vi "TidyOverlappingWires.vi"(8 "Error In":errorcluster, 10 "New case structure ref":refnum<vi>, 11 "VI ref in":refnum<vi>) -> (0 "Error Out":errorcluster)   [LabVIEW 2017, in "ErrorStructureDrawer.lvlib"]
doc: "Clean wires that are at risk of overlapping others as a result of the actions of the plugin.\n\nNote that this acts on wires that this VI thinks are \"at risk\" of overlap as there is no obvious method to directly check if wires overlap."
uses:
  ErrorStructureDrawer.lvlib
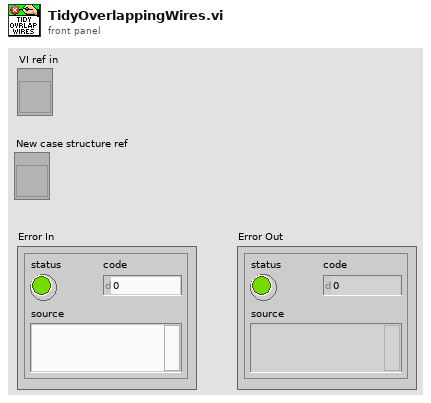
[diagram p1: front panel]
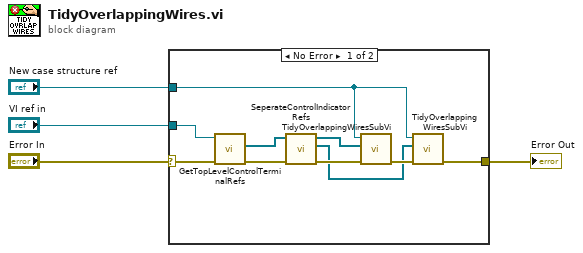
[diagram p0: block diagram]
diagram:
  n1 = case shown="No Error" "Error In" {
    selector: "Error In" -> [w6 w15]
    tunnel: "VI ref in" -> [w11 _]
    tunnel: "New case structure ref" -> [w9 _]
    tunnel: [w5 w15] -> w1
    frame No Error {
      n2 = call "GetTopLevelControlTerminalRefs.vi"("error in (no error)"=w6, "VI ref in"=w11) -> ("error out"=w13:errorcluster, "Control terminals on top-level"=w14:refnum<vi>[])  [unwired: 7 in, 1 out]
      n3 = call "SeperateControlIndicatorRefs.vi"("error in (no error)"=w13, "Terminal references"=w14) -> ("error out"=w12:errorcluster, "Indicator references"=w7:refnum<vi>[], "Control references"=w10:refnum<vi>[])  [unwired: 7 in]
      n4 = call "TidyOverlappingWiresSubVi.vi"("Error In"=w12, "Control references"=w10, "New case structure ref"=w9) -> ("Error Out"=w8:errorcluster)  [unwired: 8 in]
      n5 = call "TidyOverlappingWiresSubVi.vi"("Error In"=w8, "Control references"=w7, "New case structure ref"=w9) -> ("Error Out"=w5:errorcluster)  [unwired: 8 in]
    }
    frame Error {
    }
  }
  "Error Out" <- w1
